vi "PlungeMap.vi"(10 "Scaling?":u16(ring) items=["Medium", "Large", "Small"], 11 "Input (pA)":dbl) -> (3 "output":dbl)   [LabVIEW 2019]
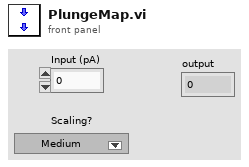
[diagram p1: front panel]
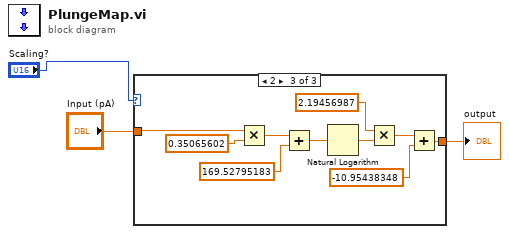
[diagram p0: block diagram]
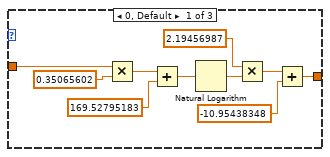
[diagram p2: hidden frame]
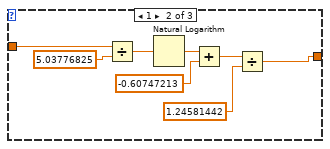
[diagram p3: hidden frame]
diagram:
  n1 = case shown="2" "Scaling?" {
    tunnel: "Input (pA)" -> [w5 w21 w24]
    tunnel: [w4 w16 w23] -> w2
    frame 0, Default {
      n2 = Multiply(x=w5, y=0.35065602) -> (x*y=w12:dbl)
      n3 = Add(x=w12, y=169.52795183) -> (x+y=w10:dbl)
      n4 = Natural Logarithm(1:w10) -> (0:w9:dbl)
      n5 = Multiply(x=2.19456987, y=w9) -> (x*y=w7:dbl)
      n6 = Add(x=w7, y=-10.95438348) -> (x+y=w4:dbl)
    }
    frame 1 {
      n7 = Divide(x=w21, y=5.03776825) -> (x/y=w19:dbl)
      n8 = Natural Logarithm(1:w19) -> (0:w18:dbl)
      n9 = Add(x=w18, y=-0.60747213) -> (x+y=w17:dbl)
      n10 = Divide(x=w17, y=1.24581442) -> (x/y=w16:dbl)
    }
    frame 2 {
      n11 = Multiply(x=w24, y=0.35065602) -> (x*y=w30:dbl)
      n12 = Add(x=w30, y=169.52795183) -> (x+y=w28:dbl)
      n13 = Natural Logarithm(1:w28) -> (0:w27:dbl)
      n14 = Multiply(x=2.19456987, y=w27) -> (x*y=w26:dbl)
      n15 = Add(x=w26, y=-10.95438348) -> (x+y=w23:dbl)
    }
  }
  "output" <- w2
